vi "Temperature warnings.vi"() -> ()   [LabVIEW 2015]
doc: "Inputs: current temperature\nOutputs: Warnings"
panel:
  out "Warning?":bool
  out "Warning Text":string
  in  "Min Temperature":dbl
  in  "Max Temperature":dbl
  in  "Current Temperature":dbl
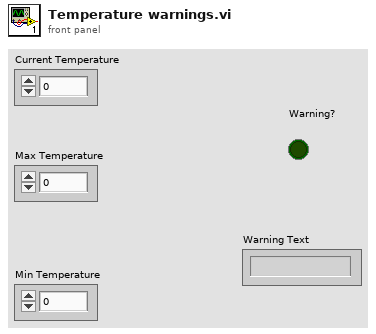
[diagram p1: front panel]
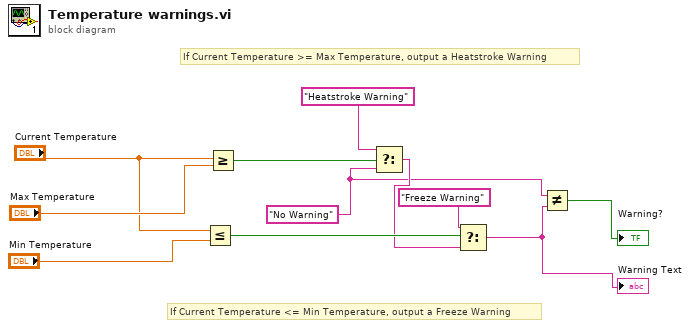
[diagram p0: block diagram]
diagram:
  w3 = "No Warning"
  # "If Current Temperature <= Min Temperature, output a Freeze Warning"
  # "If Current Temperature >= Max Temperature, output a Heatstroke Warning"
  n1 = Less Or Equal?(x="Current Temperature", y="Min Temperature") -> (x <= y?=w6:bool)
  n2 = Greater Or Equal?(x="Current Temperature", y="Max Temperature") -> (x >= y?=w8:bool)
  n3 = Select(t="Heatstroke Warning", s=w8, f=w3) -> (s? t:f=w4:string)
  n4 = Select(t="Freeze Warning", s=w6, f=w4) -> (s? t:f=w1:string)
  "Warning Text" <- w1
  n5 = Not Equal?(x=w3, y=w1) -> (x != y?=→"Warning?":bool)
